vi "CellClick Event Callback2.vi"(4 "User Parameter":variant, 5 "Event Data":cluster{"sender":refnum<k24>, "e":refnum<k24>}, 6 "Control Ref":refnum<k24>, 7 "Event Common Data":T1) -> ()   [LabVIEW 2014]
uses:
  System.Windows.Forms
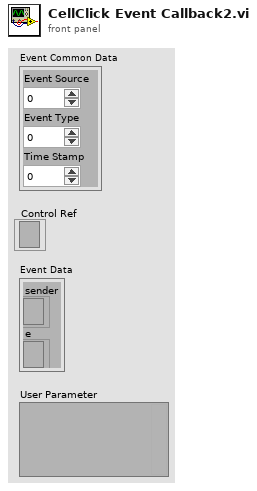
[diagram p1: front panel]
types:
  T1 = cluster{"Event Source":i32, "Event Type":u32, "Time Stamp":u32}
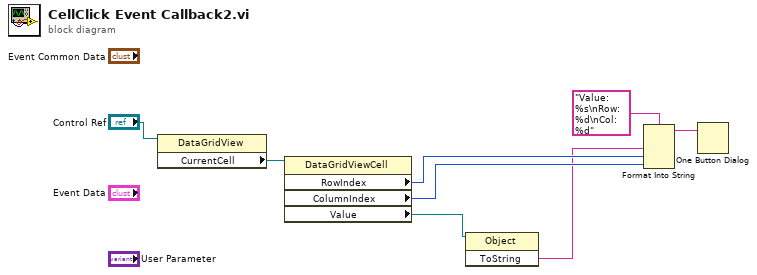
[diagram p0: block diagram]
diagram:
  n1 = property class="DataGridView"(reference="Control Ref") -> ("CurrentCell"=w7:refnum<k24>)  [unwired: 1 in, 2 out]
  n2 = property class="DataGridViewCell"(reference=w7) -> ("RowIndex"=w5:i32, "ColumnIndex"=w4:i32, "Value"=w1:refnum<k24>)  [unwired: 1 in, 2 out]
  n3 = invoke class="Object" method="ToString"(reference=w1) -> ("ToString"=w2:string)  [unwired: 2 in, 2 out]
  n4 = Format Into String(format string="Value: %s\nRow: %d\nCol: %d", w2, w5, w4) -> (resulting string=w6:string)  [unwired: 2 in, 1 out]
  n5 = One Button Dialog(message=w6) -> ()  [unwired: 1 in, 1 out]
